vi "1B spoof drag.vi"(6 "time elapsed since last iteration":dbl, 7 "Hull Drag Coefficient":dbl=0.05, 9 "Speed":dbl, 10 "Rudder Drag Coefficient":dbl=0.05, 11 "Rudder Angle":T1) -> (2 "Total Drag dV":dbl, 3 "Rudder Drag":dbl)   [LabVIEW 2011]
doc: "Calculates the hydrodynamic drag force on the boat. Drag force has two components: \n1. hull drag, which is proportional to a fixed hull drag coefficient and the square of the boat speed, and\n2. rudder drag, which is proportional to a rudder drag coefficient, the amount of rudder surface as viewed from the front of the boat (sine of rudder angle), and the square of the boat speed.\nby Jason"
uses:
  2-Think/2 Typedefs/rudder angle.ctl
panel:
  out "Boolean 3":bool
  out "Boolean 2":bool
  out "Drag too big?":bool
  # "quirk: large timesteps sometimes made a drag dV greater\nthan the total velocity, making the boat go backwards.\nI added this coercion to make sure drag doesn't push\nthe boat past 0 velocity."
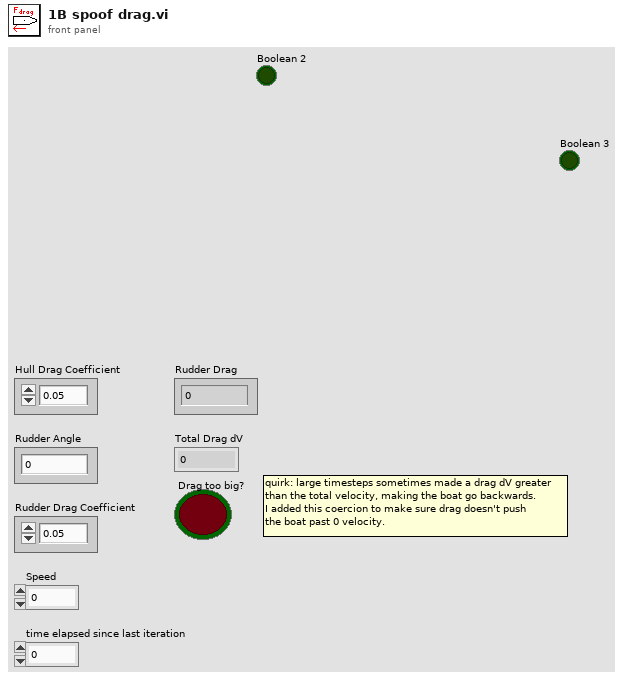
[diagram p1: front panel]
types:
  T1 = typedef "rudder angle.ctl" = dbl
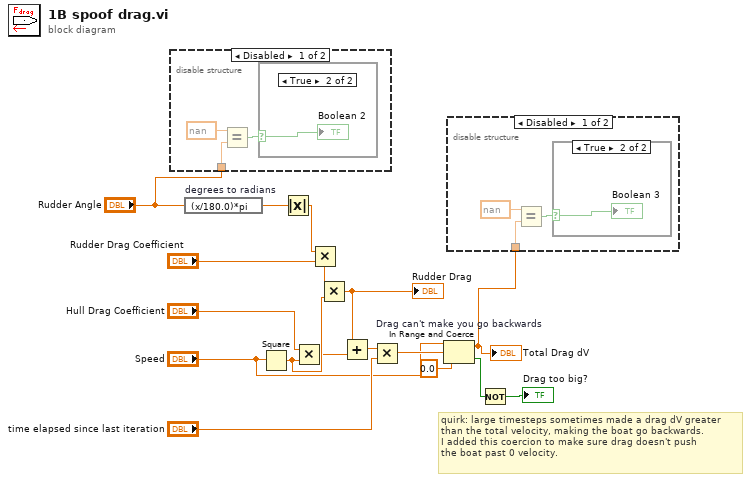
[diagram p0: block diagram]
diagram:
  # "quirk: large timesteps sometimes made a drag dV greater\nthan the total velocity, making the boat go backwards.\nI added this coercion to make sure drag doesn't push\nthe boat past 0 velocity."
  n1 = disable-structure shown="Disabled" {
    disable-tunnel: "Rudder Angle" -> [w18 _]
    frame Disabled {
      n2 = Equal?(x=nan, y=w18) -> (x = y?=w20:bool)
      n3 = case shown="True" w20 {
        selector: w20 -> [_ w21]
        frame False {
        }
        frame True {
          "Boolean 2" <- w21
        }
      }
    }
    frame Enabled {
    }
  }
  n4 = expression code="(x/180.0)*pi" "degrees to radians"("Rudder Angle") -> (w2:T1)
  n5 = Square(x="Speed") -> (x^2=w14:dbl)
  n6 = Absolute Value(x=w2) -> (abs(x)=w12:T1)
  n7 = Multiply(x="Hull Drag Coefficient", y=w14) -> (x*y=w11:dbl)
  n8 = Multiply(x=w12, y="Rudder Drag Coefficient") -> (x*y=w13:T1)
  n9 = Multiply(x=w13, y=w14) -> (x*y=w15:T1)
  "Rudder Drag" <- w15
  n10 = Add(x=w15, y=w11) -> (x+y=w16:T1)
  n11 = Multiply(x=w16, y="time elapsed since last iteration") -> (x*y=w8:T1)
  n12 = In Range and Coerce "Drag can't make you go backwards"(upper limit="Speed", x=w8, lower limit=0.0) -> (coerced(x)=w4:T1, In Range?=w7:bool)
  "Total Drag dV" <- w4
  n13 = disable-structure shown="Disabled" {
    disable-tunnel: w4 -> [w22 _]
    frame Disabled {
      n14 = Equal?(x=nan, y=w22) -> (x = y?=w24:bool)
      n15 = case shown="True" w24 {
        selector: w24 -> [_ w25]
        frame False {
        }
        frame True {
          "Boolean 3" <- w25
        }
      }
    }
    frame Enabled {
    }
  }
  n16 = Not(x=w7) -> (.not. x?=→"Drag too big?":bool)
